vi "Acquisition Message Loop.vi"(8 "error in (no error)":errorcluster, 9 "queue out":refnum<queue>, 10 "Data Notifier":refnum<notifier>, 11 "Message Queues":T1) -> (0 "error out":errorcluster)   [LabVIEW 2018, in "Acquisition.lvlib"]
doc: "Message loop for handling messages pertaining to the acquisition of data from the hardware."
uses:
  Acquisition.lvlib
  support/Message Queue/Message Queue.lvlib
  Acquisition State.ctl
  support/Message Queue/Enqueue Message (Single).vi
  <vilib>/ErrorRing/Error Ring.xnode
  GlobalVariable/GlobalPowerByTime.vi
  GlobalVariable/Globalt0.vi
  GlobalVariable/GlobalLongueurOnde.vi
  GlobalVariable/GlobalDisconnected.vi
  GlobalVariable/GlobalPosXbyTime.vi
  GlobalVariable/GlobalPosYbyTime.vi
  GlobalVariable/GlobalProfileByTime.vi
  GlobalVariable/GlobalTimeStep.vi
  GlobalVariable/GlobalFirstRep.vi
  GlobalVariable/GlobalTensionByTime.vi
  GlobalVariable/GlobalTemperatureByTime.vi
  <vilib>/Utility/error.llb/Error Cluster From Error Code.vi
  support/Message Queue/Message Cluster.ctl
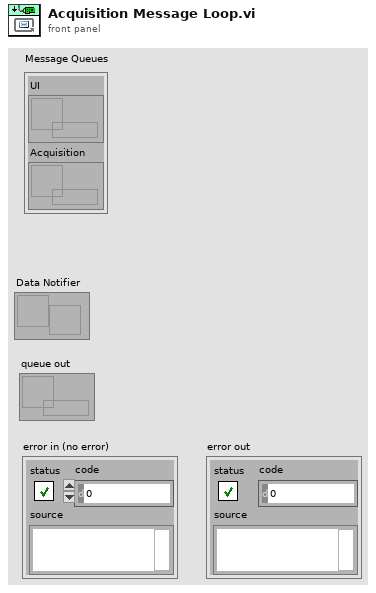
[diagram p1: front panel]
types:
  T1 = cluster{"UI":refnum<queue>, "Acquisition":refnum<queue>}
  T2 = typedef "Acquisition.lvlib/Acquisition State.ctl" = enum16{"Idle", "Acquiring"}
  T3 = enum16{"open", "replace", "create", "open or create", "replace or create", "replace or create with confirmation"}
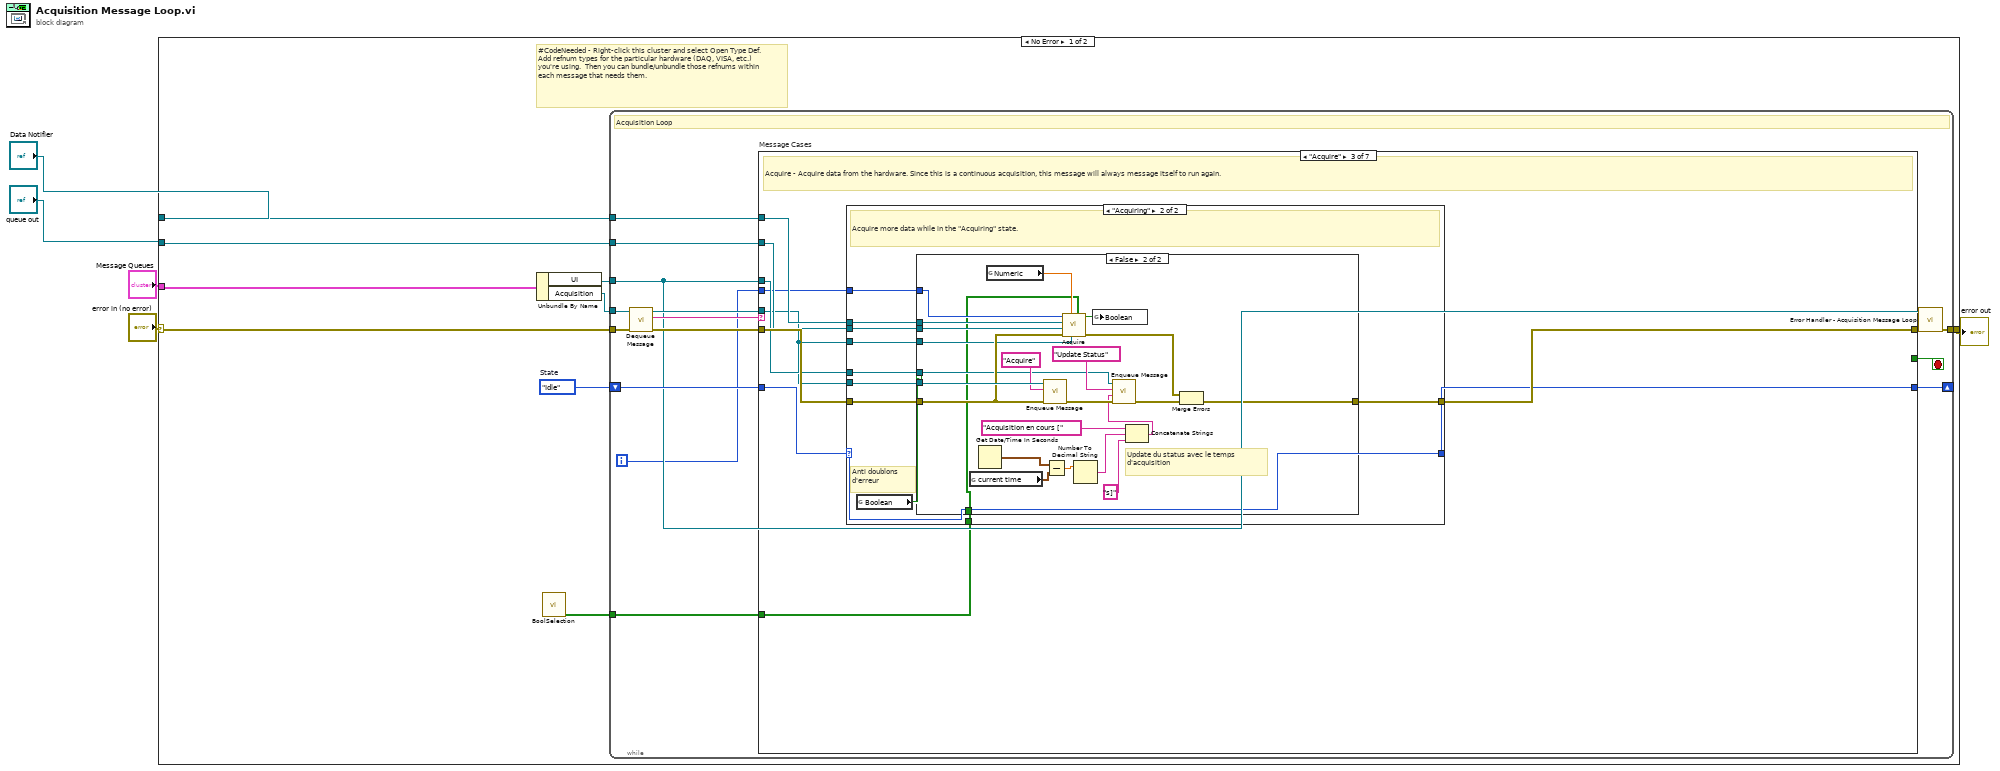
[diagram p0: block diagram]
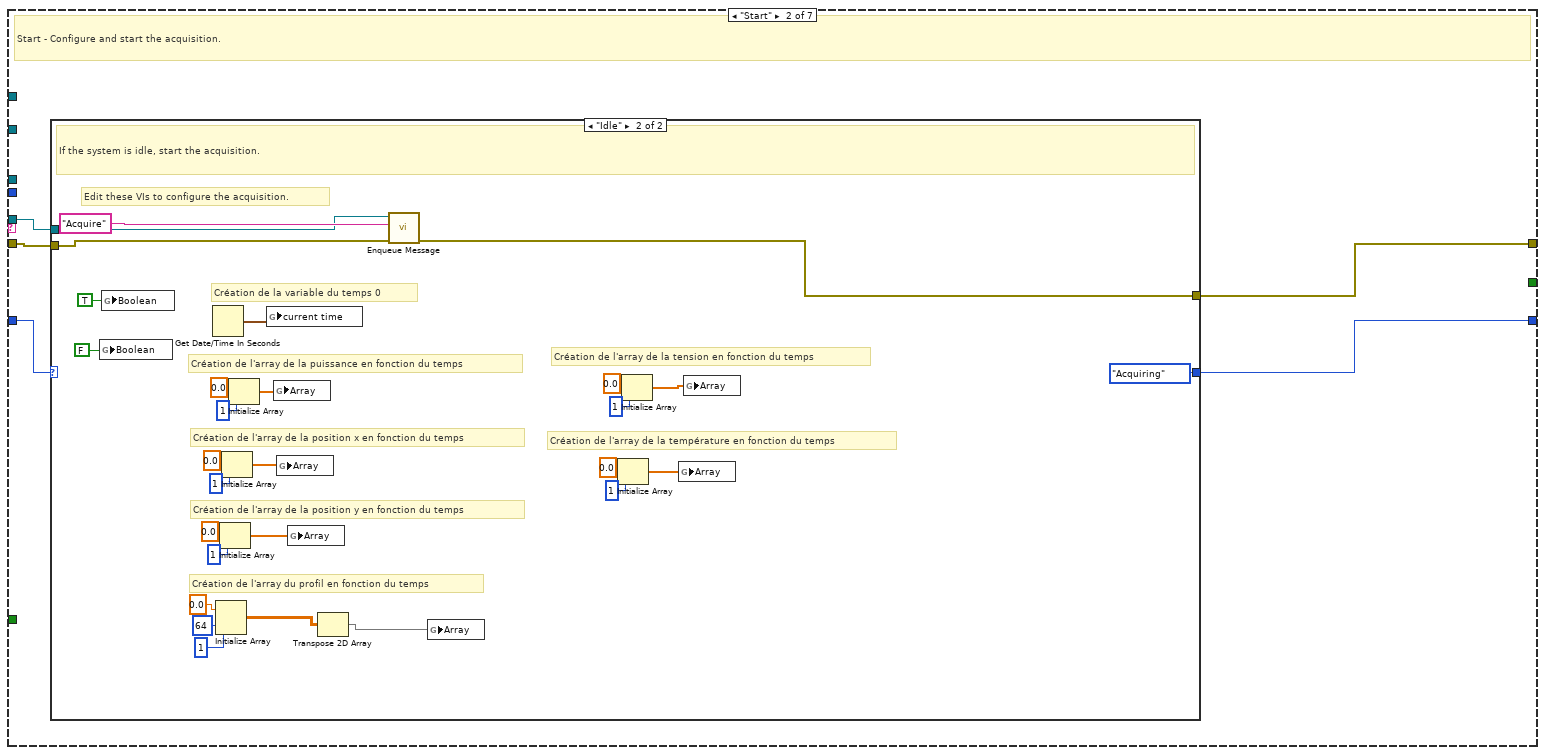
[diagram p3: hidden frame]
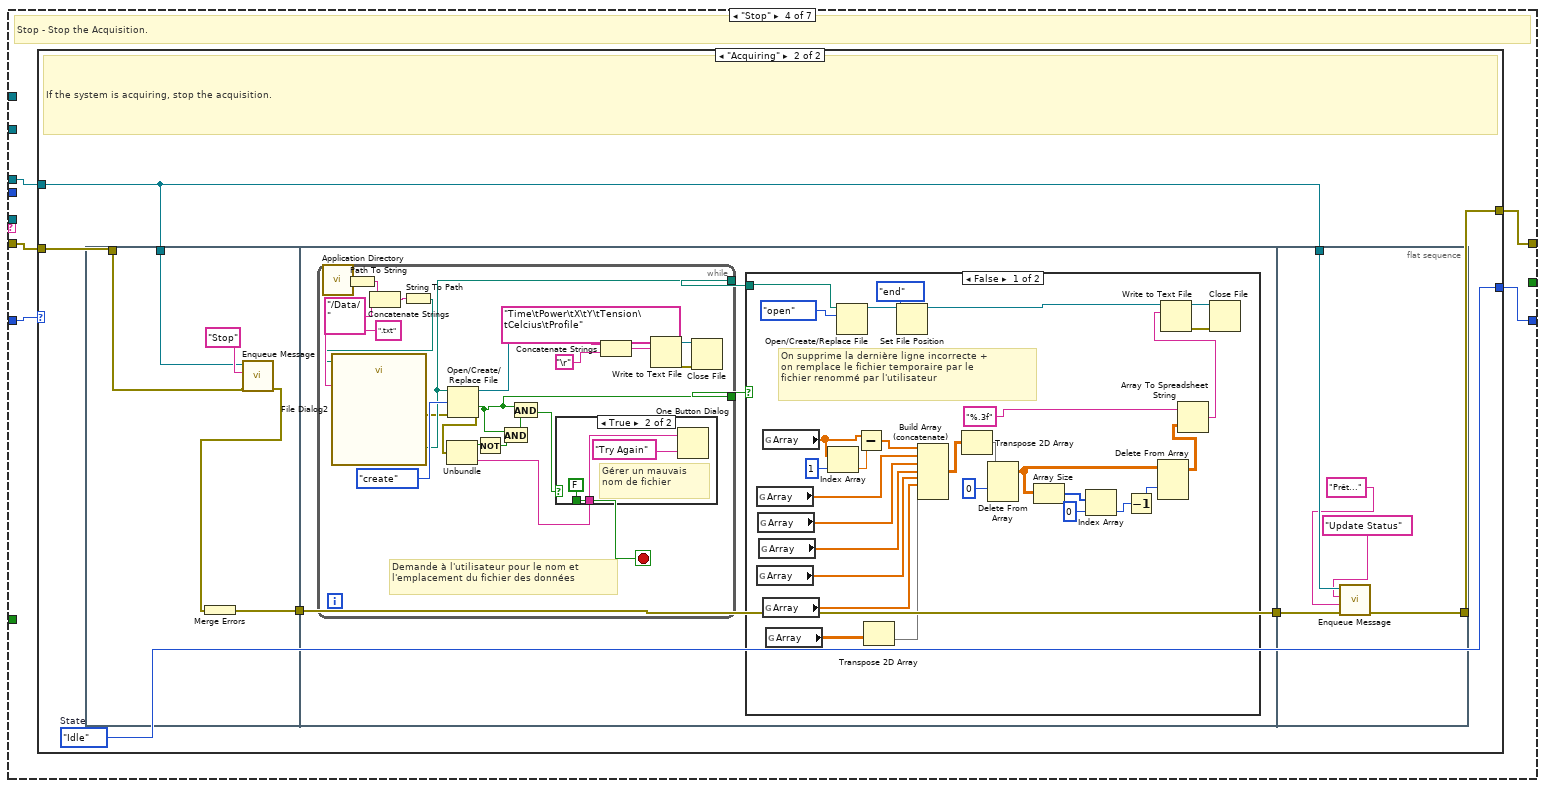
[diagram p7: hidden frame]
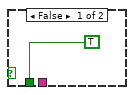
[diagram p10: hidden frame]
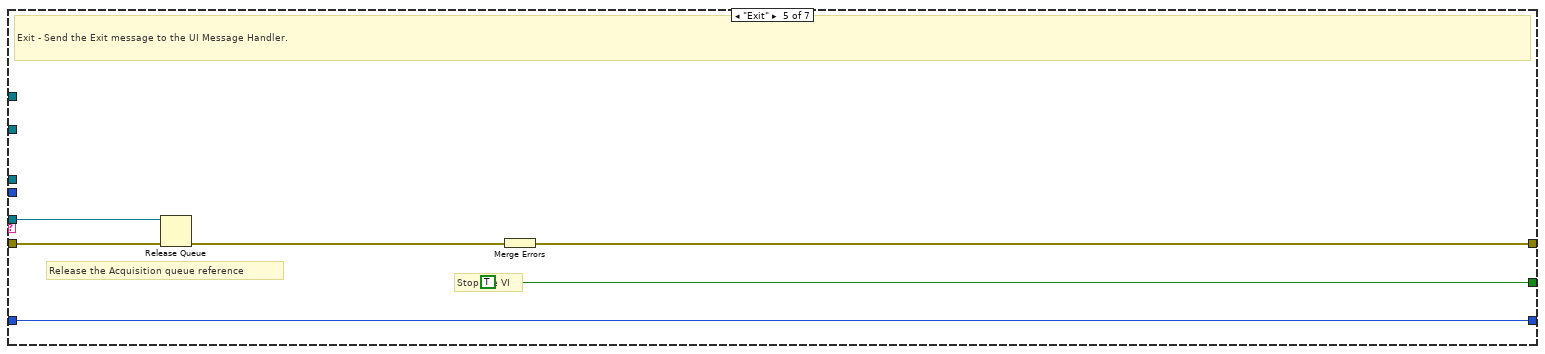
[diagram p11: hidden frame]
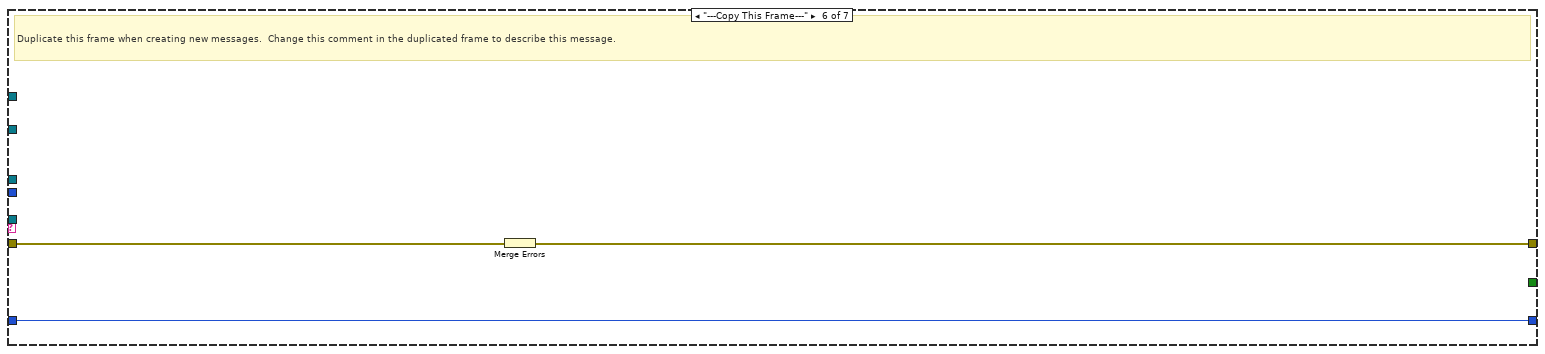
[diagram p12: hidden frame]
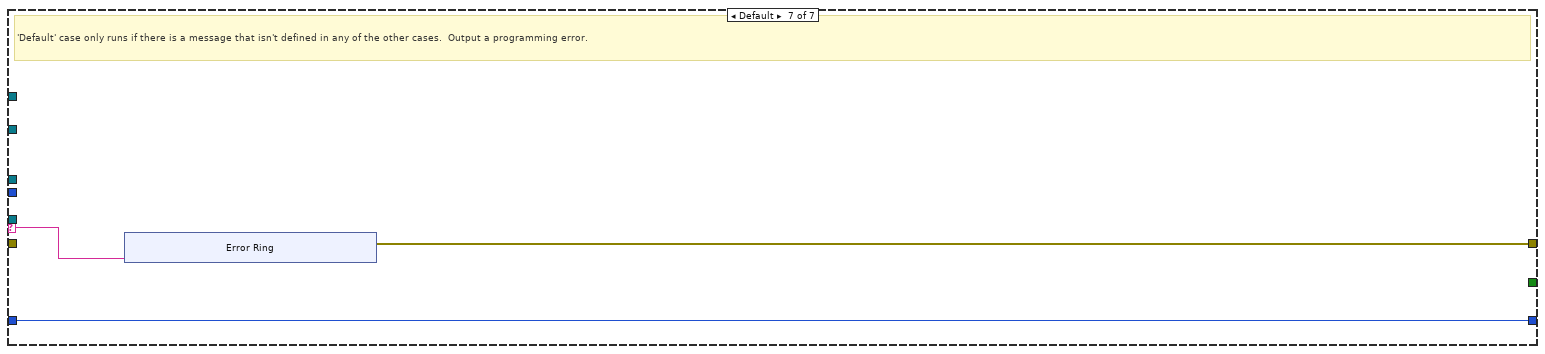
[diagram p13: hidden frame]
diagram:
  n1 = case shown="No Error" "error in (no error)" {
    selector: "error in (no error)" -> [w11 w215]
    tunnel: "Message Queues" -> [w14 _]
    tunnel: [w12 w215] -> w4
    tunnel: "Data Notifier" -> [w9 _]
    tunnel: "queue out" -> [w8 _]
    frame No Error {
      w7 = Acquisition_State."Idle"  # State
      # "#CodeNeeded - Right-click this cluster and select Open Type Def.  Add refnum types for the particular hardware (DAQ, VISA, etc.) you're using.  Then you can bundle/unbundle those refnums within each message that needs them."
      n2 = Unbundle By Name(w14) -> ("UI"=w10:refnum<queue>, "Acquisition"=w13:refnum<queue>)
      n3 = call "BoolSelection.vi"() -> ("BoolSelection"=w6:bool[][])  [unwired: 11 in]
      n4 = while {
        tunnel: w13 -> [w17]
        tunnel: w10 -> [w18]
        tunnel: w9 -> [w25]
        tunnel: w8 -> [w24]
        shift-right: [w22] -> _
        shift-left: w7 -> [w23]
        tunnel: w11 -> [w28]
        tunnel: [w21] -> w12
        tunnel: w6 -> [w15]
        i -> [w16]
        stop <- w29 stop-if-true
        # "Acquisition Loop"
        n5 = call "Dequeue Message.vi"("error in (no error)"=w28, "Message Queue"=w17) -> ("error out"=w27:errorcluster, "Message"=w26:string, "dup Message Queue"=w19:refnum<queue>)  [unwired: 6 in, 1 out]
        n6 = case "Message Cases" shown="\"Acquire\"" w26 {
          selector: w26 -> [_ _ _ _ _ _ w205]
          tunnel: w19 -> [_ w34 w69 _ w197 _ _]
          tunnel: w27 -> [w31 w35 w75 w117 w199 w204 _]
          tunnel: [w31 w36 w76 w115 w200 w203 w206] -> w20
          tunnel: [_ _ _ _ TRUE _ _] -> w29
          tunnel: w18 -> [_ _ w70 w116 _ _ _]
          tunnel: w25 -> [_ _ w74 _ _ _ _]
          tunnel: w24 -> [_ _ w73 _ _ _ _]
          tunnel: w23 -> [w30 w32 w71 w118 w196 w202 w207]
          tunnel: [w30 w33 w72 w114 w196 w202 w207] -> w22
          tunnel: w16 -> [_ _ w68 _ _ _ _]
          tunnel: w15 -> [_ _ w67 _ _ _ _]
          frame "Initialize" {
            # "Initialize  - Initialize is currently a no-op.  The hardware initialization takes place in the 'Start' message."
          }
          frame "Start" {
            # "Start - Configure and start the acquisition."
            n7 = case shown="\"Idle\"" w32 {
              selector: w32 -> [w37 _]
              tunnel: [w38 w62] -> w36
              tunnel: w35 -> [w38 w66]
              tunnel: w34 -> [_ w63]
              tunnel: [w37 Acquisition_State."Acquiring" ("Acquisition State")] -> w33
              frame "Acquiring" {
                # "The system is already acquiring. Ignore the \"Start\" message."
              }
              frame "Idle" {
                # "Création de l'array de la température en fonction du temps"
                # "Création de l'array de la tension en fonction du temps"
                # "Création de la variable du temps 0"
                # "Création de l'array du profil en fonction du temps"
                # "Création de l'array de la position y en fonction du temps"
                # "Création de l'array de la position x en fonction du temps"
                # "Création de l'array de la puissance en fonction du temps"
                # "Edit these VIs to configure the acquisition."
                # "If the system is idle, start the acquisition."
                n8 = global write "GlobalDisconnected.vi" "Boolean"(FALSE) -> ()
                n9 = global write "GlobalFirstRep.vi" "Boolean"(TRUE ("Boolean")) -> ()
                n10 = Get Date/Time In Seconds() -> (seconds since 1Jan1904=w45:timestamp)
                n11 = Initialize Array(0.0, 64 ("dimension size"), 1 ("dimension size")) -> (w58:dbl[][])
                n12 = Initialize Array(0.0, 1) -> (w59:dbl[])
                n13 = Initialize Array(0.0, 1) -> (w60:dbl[])
                n14 = Initialize Array(0.0, 1) -> (w61:dbl[])
                n15 = global write "Globalt0.vi" "current time"(w45) -> ()
                n16 = global write "GlobalPowerByTime.vi" "Array"(w61) -> ()
                n17 = global write "GlobalPosXbyTime.vi" "Array"(w60) -> ()
                n18 = global write "GlobalPosYbyTime.vi" "Array"(w59) -> ()
                n19 = Transpose 2D Array(2D array=w58) -> (transposed array=w57:dbl[][])
                n20 = call-poly "Enqueue Message.vi"("error in (no error)"=w66, "Message"="Acquire", "Message Queue"=w63) -> ("error out"=w62:errorcluster)  [unwired: 7 in, 1 out]
                n21 = global write "GlobalProfileByTime.vi" "Array"(w57) -> ()
                n22 = Initialize Array(0.0, 1) -> (w39:dbl[])
                n23 = Initialize Array(0.0, 1) -> (w40:dbl[])
                n24 = global write "GlobalTemperatureByTime.vi" "Array"(w39) -> ()
                n25 = global write "GlobalTensionByTime.vi" "Array"(w40) -> ()
              }
            }
          }
          frame "Acquire" {
            # "Acquire - Acquire data from the hardware. Since this is a continuous acquisition, this message will always message itself to run again."
            n26 = case shown="\"Acquiring\"" w71 {
              selector: w71 -> [w77 w85]
              tunnel: [w78 w89] -> w76
              tunnel: w69 -> [_ w88]
              tunnel: w75 -> [w78 w84]
              tunnel: w74 -> [_ w87]
              tunnel: w73 -> [_ w86]
              tunnel: [w77 w85] -> w72
              tunnel: w70 -> [_ w83]
              tunnel: w69 -> [_ w82]
              tunnel: w68 -> [_ w80]
              tunnel: w67 -> [_ w79]
              frame "Idle" {
                # "Ignore \"Acquire\" messages when the acquisition is idle."
              }
              frame "Acquiring" {
                # "Anti doublons\nd'erreur"
                # "Acquire more data while in the \"Acquiring\" state."
                n27 = global read "GlobalDisconnected.vi" "Boolean"() -> (w81:bool)
                n28 = case shown="False" w81 {
                  tunnel: [w90 w113] -> w89
                  tunnel: w88 -> [_ w112]
                  tunnel: w87 -> [_ w109]
                  tunnel: w86 -> [_ w108]
                  tunnel: w84 -> [w90 w107]
                  tunnel: w83 -> [_ w96]
                  tunnel: w82 -> [_ w95]
                  tunnel: w80 -> [_ w92]
                  tunnel: w79 -> [_ w91]
                  frame True {
                  }
                  frame False {
                    # "Update du status avec le temps\nd'acquisition"
                    n29 = global read "Globalt0.vi" "current time"() -> (w102:timestamp)
                    n30 = Get Date/Time In Seconds() -> (seconds since 1Jan1904=w101:timestamp)
                    n31 = global read "GlobalLongueurOnde.vi" "Numeric"() -> (w94:dbl)
                    n32 = call-poly "Enqueue Message.vi"("error in (no error)"=w107, "Message"="Acquire", "Message Queue"=w112) -> ("error out"=w105:errorcluster)  [unwired: 7 in, 1 out]
                    n33 = Subtract(x=w101, y=w102) -> (x-y=w103:dbl)
                    n34 = call "Acquire.vi"("Bits"=w91, "Acquisition"=w95, "Longueur d'onde"=w94, "error in (no error)"=w107, "Data Queue"=w108, "Data Notifier"=w109, "Loop Count"=w92) -> ("error out"=w111:errorcluster, "Disconnected"=w93:bool)  [unwired: 3 in]
                    n35 = Number To Decimal String(number=w103) -> (decimal integer string=w100:string)  [unwired: 1 in]
                    n36 = global write "GlobalDisconnected.vi" "Boolean"(w93) -> ()
                    n37 = Concatenate Strings("Acquisition en cours [", w100, "s]" ("string")) -> (w98:string)
                    n38 = call-poly "Enqueue Message.vi"("error in (no error)"=w105, "Message Data"=w98, "Message"="Update Status", "Message Queue"=w96) -> ("error out"=w106:errorcluster)  [unwired: 6 in, 1 out]
                    n39 = Merge Errors(w111, w106) -> (w113:errorcluster)
                  }
                }
              }
            }
          }
          frame "Stop" {
            # "Stop - Stop the Acquisition."
            n40 = case shown="\"Acquiring\"" w118 {
              selector: w118 -> [w120 _]
              tunnel: w117 -> [w119 w125]
              tunnel: w116 -> [_ w121]
              tunnel: [w119 w124] -> w115
              tunnel: [w120 w123] -> w114
              frame "Idle" {
                # "The system is already idle. Ignore the \"Stop\" message."
              }
              frame "Acquiring" {
                w123 = Acquisition_State."Idle"  # State
                # "If the system is acquiring, stop the acquisition."
                n41 = flat-sequence {
                  tunnel: [w131] -> w126
                  tunnel: w121 -> [w128]
                  tunnel: w125 -> [w127]
                  tunnel: w126 -> [w133]
                  tunnel: [w133] -> w122
                  tunnel: [w194] -> w124
                  tunnel: w122 -> [w195]
                  tunnel: w121 -> [w193]
                  frame #0 {
                    n42 = call-poly "Enqueue Message.vi"("error in (no error)"=w127, "Message"="Stop", "Message Queue"=w128) -> ("error out"=w130:errorcluster)  [unwired: 7 in, 1 out]
                    n43 = Merge Errors(w130) -> (w131:errorcluster)
                  }
                  frame #1 {
                    n44 = while {
                      tunnel: [w181] -> w134
                      tunnel: [w171] -> w132
                      stop <- w177 stop-if-true
                      # "Demande à l'utilisateur pour le nom et\nl'emplacement du fichier des données"
                      n45 = call <vilib>:"Application Directory.vi"() -> ("Application Directory"=w184:path)
                      n46 = Path To String(path=w184) -> (string=w185:string)
                      n47 = Concatenate Strings(w185, "/Data/") -> (w186:string)
                      n48 = String To Path(string=w186) -> (path=w170:path)
                      n49 = call "File Dialog2"("start path"=w170, "pattern (all files)"=".txt") -> ("selected path"=w181:path, "error out"=w179:errorcluster)  [unwired: 10 in, 2 out]
                      n50 = Open/Create/Replace File(file path (use dialog)=w181, error in=w179, operation (0:open)=T3."create") -> (refnum out=w166:refnum<file>, cancelled=w171:bool, error out=w176:errorcluster)  [unwired: 3 in]
                      n51 = Unbundle(w176) -> ("status"=w175:bool, "source"=w178:string)  [unwired: 1 out]
                      n52 = Not(x=w175) -> (.not. x?=w174:bool)
                      n53 = And(x=w171, y=w174) -> (x .and. y?=w173:bool)
                      n54 = And(x=w171, y=w173) -> (x .and. y?=w172:bool)
                      n55 = case shown="True" w172 {
                        tunnel: w178 -> [_ w190]
                        tunnel: [TRUE FALSE] -> w177
                        frame False {
                        }
                        frame True {
                          # "Gérer un mauvais \nnom de fichier"
                          n56 = One Button Dialog(message=w190, button name ("OK")="Try Again") -> ()  [unwired: 1 out]
                        }
                      }
                      n57 = Concatenate Strings("Time\tPower\tX\tY\tTension\tCelcius\tProfile", "\r") -> (w169:string)
                      n58 = Write to Text File(file (use dialog)=w166, text=w169) -> (refnum out=w165:refnum<file>, error out=w164:errorcluster)  [unwired: 2 in, 1 out]
                      n59 = Close File(refnum=w165, error in=w164) -> ()  [unwired: 2 out]
                    }
                    n60 = case shown="False" w132 {
                      tunnel: w134 -> [w157 _]
                      frame False {
                        # "On supprime la dernière ligne incorrecte + \non remplace le fichier temporaire par le \nfichier renommé par l'utilisateur"
                        n61 = global read "GlobalPowerByTime.vi" "Array"() -> (w156:dbl[])
                        n62 = global read "GlobalTensionByTime.vi" "Array"() -> (w136:dbl[])
                        n63 = global read "GlobalPosXbyTime.vi" "Array"() -> (w155:dbl[])
                        n64 = global read "GlobalPosYbyTime.vi" "Array"() -> (w154:dbl[])
                        n65 = global read "GlobalTimeStep.vi" "Array"() -> (w144:dbl[])
                        n66 = global read "GlobalTemperatureByTime.vi" "Array"() -> (w135:dbl[])
                        n67 = global read "GlobalProfileByTime.vi" "Array"() -> (w152:dbl[][])
                        n68 = Index Array(array=w144, index=1) -> (element=w145:dbl)
                        n69 = Open/Create/Replace File(file path (use dialog)=w157, operation (0:open)=T3."open") -> (refnum out=w161:refnum<file>)  [unwired: 4 in, 2 out]
                        n70 = Subtract(x=w144, y=w145) -> (x-y=w143:dbl[])
                        n71 = Transpose 2D Array(2D array=w152) -> (transposed array=w151:dbl[][])
                        n72 = Set File Position(refnum=w161, from (0:start)=enum16{"start", "end", "current"}."end") -> (refnum out=w163:refnum<file>)  [unwired: 2 in, 1 out]
                        n73 = Build Array (concatenate)(w143, w156, w155, w154, w136, w135, w151) -> (w153:dbl[][])
                        n74 = Transpose 2D Array(2D array=w153) -> (transposed array=w147:dbl[][])
                        n75 = Delete From Array(array=w147, index (row)=0) -> (array with subset deleted=w138:dbl[][])  [unwired: 2 in, 1 out]
                        n76 = Array Size(array=w138) -> (size(s)=w142:i32[])
                        n77 = Index Array(array=w142, index=0) -> (element=w140:i32)
                        n78 = Decrement(x=w140) -> (x-1=w139:i32)
                        n79 = Delete From Array(array=w138, index (row)=w139) -> (array with subset deleted=w137:dbl[][])  [unwired: 2 in, 1 out]
                        n80 = Array To Spreadsheet String(array=w137, 3:"%.3f" ("format string")) -> (spreadsheet string=w162:string)  [unwired: 1 in]
                        n81 = Write to Text File(file (use dialog)=w163, text=w162) -> (refnum out=w150:refnum<file>, error out=w149:errorcluster)  [unwired: 2 in, 1 out]
                        n82 = Close File(refnum=w150, error in=w149) -> ()  [unwired: 2 out]
                      }
                      frame True {
                      }
                    }
                  }
                  frame #2 {
                    n83 = call-poly "Enqueue Message.vi"("error in (no error)"=w195, "Message Data"="Prêt...", "Message"="Update Status", "Message Queue"=w193) -> ("error out"=w194:errorcluster)  [unwired: 6 in, 1 out]
                  }
                }
              }
            }
          }
          frame "Exit" {
            # "Release the Acquisition queue reference"
            # "Stop the VI"
            # "Exit - Send the Exit message to the UI Message Handler."
            n84 = Release Queue(queue=w197, error in (no error)=w199) -> (error out=w198:errorcluster)  [unwired: 1 in, 2 out]
            n85 = Merge Errors(w198) -> (w200:errorcluster)
          }
          frame "---Copy This Frame---" {
            # "Duplicate this frame when creating new messages.  Change this comment in the duplicated frame to describe this message."
            n86 = Merge Errors(w204) -> (w203:errorcluster)
          }
          frame Default {
            # "'Default' case only runs if there is a message that isn't defined in any of the other cases.  Output a programming error."
            n87 = xnode "Error Ring"("parameter 0"=w205) -> ("error out"=w206:errorcluster)
          }
        }
        n88 = call "Error Handler - Acquisition Message Loop.vi"("error in (no error)"=w20, "Message Queue"=w18) -> ("dup error in"=w21:errorcluster)  [unwired: 8 in, 1 out]
      }
    }
    frame Error {
    }
  }
  "error out" <- w4
